vi "ExProg_ParseFromScript.vi"(11 "text":string) -> (1 "error?":bool, 2 "program":T1[](array[typedef]))   [LabVIEW 2011]
uses:
  ExProgCommandType.ctl
  ExProgCommandEnumType.ctl
  Motors/MotorAxisEnum.ctl
panel:
  in  "Command":T1={"cmd"=enum."wait", "axis"=enum."magrot", "value/pos"=0.0, "speed"=0.0, "name"=""}
  # "(used for commands with string parameters)"
  # "(used for commands with string parameters)"
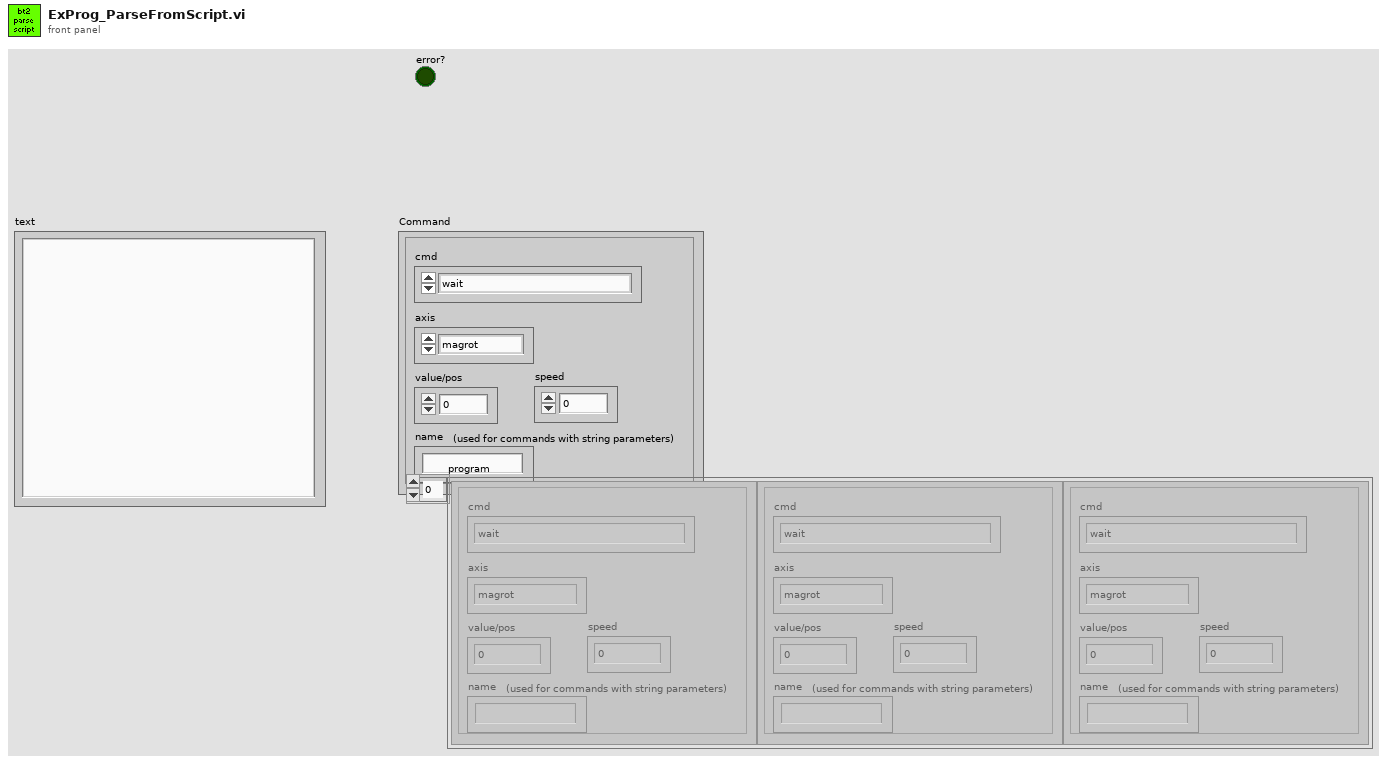
[diagram p1: front panel]
types:
  T1 = typedef "ExProgCommandType.ctl" = cluster{"cmd":T2, "axis":T3, "value/pos":dbl, "speed":dbl, "name":string}
  T2 = typedef "ExProgCommandEnumType.ctl" = enum16{"wait", "move", "event", "idle", "when", "section", "stop"}
  T3 = typedef "MotorAxisEnum.ctl" = enum16{"no axis", "magrot", "magpos", "px", "py", "pz", "camx", "camy"}
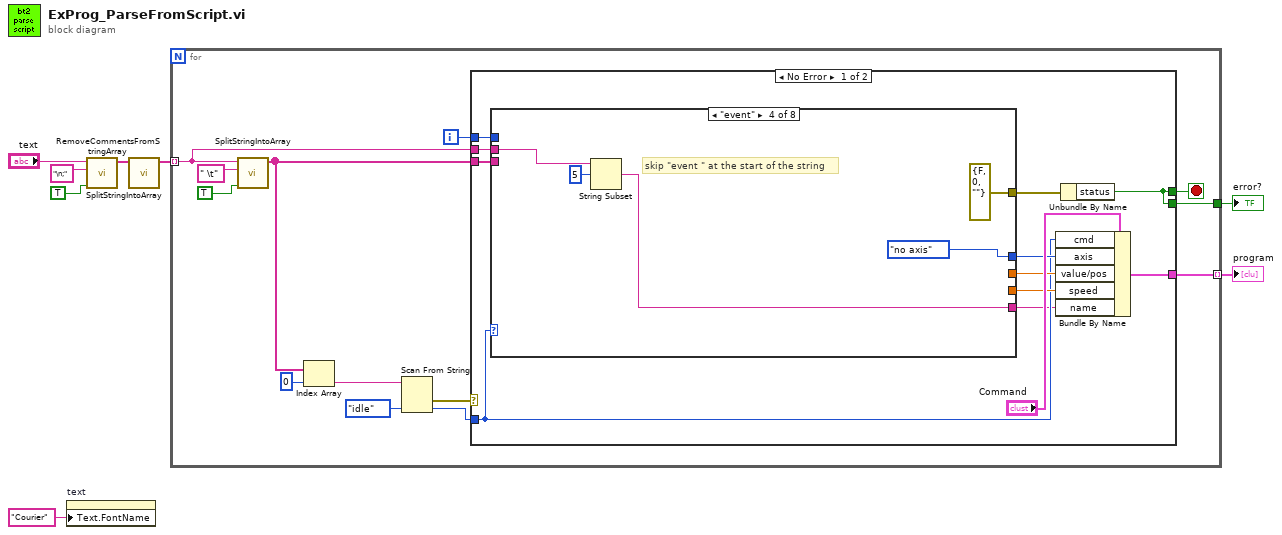
[diagram p0: block diagram]
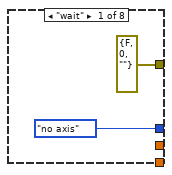
[diagram p2: hidden frame]
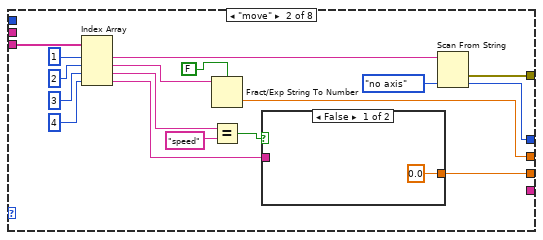
[diagram p3: hidden frame]
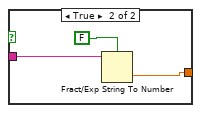
[diagram p4: hidden frame]
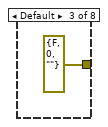
[diagram p5: hidden frame]
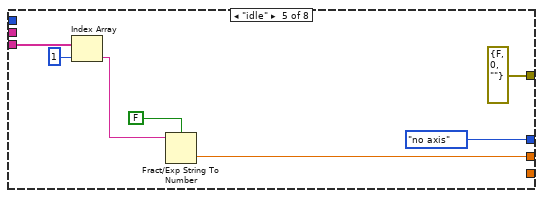
[diagram p6: hidden frame]
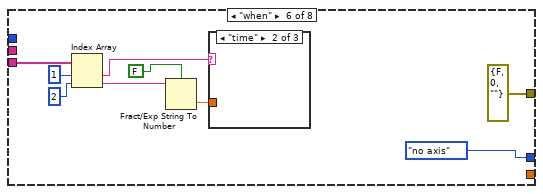
[diagram p7: hidden frame]
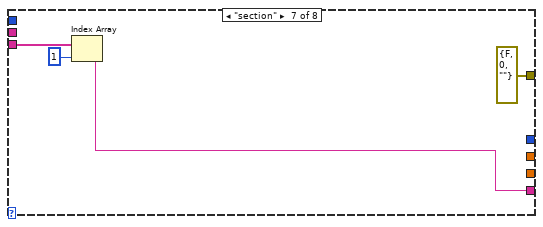
[diagram p10: hidden frame]
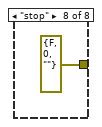
[diagram p11: hidden frame]
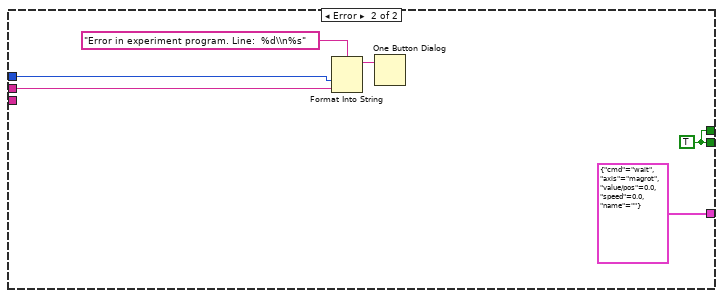
[diagram p12: hidden frame]
diagram:
  n1 = property on="text" class="Str"("Text.FontName"="Courier" ("Text.Font:Name")) -> ()  [unwired: 2 in, 2 out]
  n2 = call "SplitStringIntoArray.vi"("remove empty entries? (F)"=TRUE, "seperators"="\n;" ("seperator"), "text"="text") -> ("result"=w3:string[])  [unwired: 7 in, 1 out]
  n3 = call "RemoveCommentsFromStringArray.vi"("input text"=w3) -> ("output array"=w2:string[])  [unwired: 10 in]
  n4 = for {
    tunnel: w2 -> [w11] mode=indexing
    tunnel: [w20] -> w5 mode=indexing
    tunnel: [w9] -> w1
    i -> [w14]
    stop <- w12 stop-if-true
    n5 = call "SplitStringIntoArray.vi"("remove empty entries? (F)"=TRUE, "seperators"=" \t", "text"=w11) -> ("result"=w15:string[])  [unwired: 7 in, 1 out]
    n6 = Index Array(array=w15, index=0) -> (element=w18:string)
    n7 = Scan From String(input string=w18, default 1=ExProgCommandEnumType."idle" ("cmd")) -> (error out=w13:errorcluster, output 1=w16:T2)  [unwired: 3 in, 2 out]
    n8 = case shown="No Error" w13 {
      tunnel: [w32 T1 {"cmd"=enum."wait", "axis"=enum."magrot", "value/pos"=0.0, "speed"=0.0, "name"=""} ("Command")] -> w20
      tunnel: w16 -> [w24 _]
      tunnel: w15 -> [w31 _]
      tunnel: w14 -> [w29 w86]
      tunnel: [w25 w84] -> w12
      tunnel: w11 -> [w22 w85]
      tunnel: [w25 w84] -> w9
      frame No Error {
        n9 = case shown="\"event\"" w24 {
          tunnel: w31 -> [_ w52 _ _ w69 w78 w82 _]
          tunnel: [_ w47 _ _ w65 _ _ _] -> w30
          tunnel: w29 -> [_ _ _ _ _ _ _ _]
          tunnel: [_ w42 _ _ _ _ _ _] -> w28
          tunnel: [MotorAxisEnum."no axis" ("Motor Axis") w37 _ MotorAxisEnum."no axis" ("Motor Axis") MotorAxisEnum."no axis" ("Motor Axis") MotorAxisEnum."no axis" ("Motor Axis") _ _] -> w27
          tunnel: [errorcluster {"status"=FALSE, "code"=0, "source"=""} ("error IO") w36 errorcluster {"status"=FALSE, "code"=0, "source"=""} ("error IO") errorcluster {"status"=FALSE, "code"=0, "source"=""} ("error IO") errorcluster {"status"=FALSE, "code"=0, "source"=""} ("error IO") errorcluster {"status"=FALSE, "code"=0, "source"=""} ("error IO") errorcluster {"status"=FALSE, "code"=0, "source"=""} ("error IO") errorcluster {"status"=FALSE, "code"=0, "source"=""} ("error IO")] -> w26
          tunnel: [_ _ _ w58 _ _ w80 _] -> w23
          tunnel: w22 -> [_ _ _ w60 _ _ _ _]
          frame "wait" {
          }
          frame "move" {
            n10 = Index Array(array=w52, index #1=1 ("index"), index #2=2 ("index"), index #3=3 ("index"), index #4=4 ("index")) -> (element #1=w39:string, element #2=w49:string, element #3=w45:string, element #4=w40:string)
            n11 = Fract/Exp String To Number(use system decimal point (T)=FALSE, string=w49) -> (number=w47:dbl)  [unwired: 2 in, 1 out]
            n12 = Equal?(x=w45, y="speed") -> (x = y?=w43:bool)
            n13 = case shown="False" w43 {
              tunnel: [0.0 w55] -> w42
              tunnel: w40 -> [_ w56]
              frame False {
              }
              frame True {
                n14 = Fract/Exp String To Number(use system decimal point (T)=FALSE, string=w56) -> (number=w55:dbl)  [unwired: 2 in, 1 out]
              }
            }
            n15 = Scan From String(input string=w39, default 1=MotorAxisEnum."no axis" ("Motor Axis")) -> (error out=w36:errorcluster, output 1=w37:T3)  [unwired: 3 in, 2 out]
          }
          frame Default {
          }
          frame "event" {
            # "skip \"event \" at the start of the string"
            n16 = String Subset(string=w60, offset (0)=5) -> (substring=w58:string)  [unwired: 1 in]
          }
          frame "idle" {
            n17 = Index Array(array=w69, index=1) -> (element=w67:string)
            n18 = Fract/Exp String To Number(use system decimal point (T)=FALSE, string=w67) -> (number=w65:dbl)  [unwired: 2 in, 1 out]
          }
          frame "when" {
            n19 = Index Array(array=w78, index #1=1 ("index"), index #2=2 ("index")) -> (element #1=w76:string, element #2=w73:string)
            n20 = Fract/Exp String To Number(use system decimal point (T)=FALSE, string=w73) -> (number=w72:dbl)  [unwired: 2 in, 1 out]
            n21 = case shown="\"time\"" w76 {
              tunnel: w72 -> [_ _ _]
              frame Default {
              }
              frame "time" {
              }
              frame "frame" {
              }
            }
          }
          frame "section" {
            n22 = Index Array(array=w82, index=1) -> (element=w80:string)
          }
          frame "stop" {
          }
        }
        n23 = Bundle By Name(cluster="Command", "cmd"=w24, "axis"=w27, "value/pos"=w30, "speed"=w28, "name"=w23) -> (w32:T1)
        n24 = Unbundle By Name(w26) -> ("status"=w25:bool)
      }
      frame Error {
        w84 = TRUE
        n25 = Format Into String(format string="Error in experiment program. Line:  %d\\n%s" ("message"), w86, w85) -> (resulting string=w87:string)  [unwired: 2 in, 1 out]
        n26 = One Button Dialog(message=w87) -> ()  [unwired: 1 in, 1 out]
      }
    }
  }
  "program" <- w5
  "error?" <- w1
